vi "Collection.Dialog.vi"(8 "error in (no error)":errorcluster, 9 "ID":u16=1 min=1 format="%.0x", 10 "Existing PIDs":string[](array[string]), 11 "Name":string) -> (0 "error out":errorcluster, 1 "ID out":u16, 2 "Cancel PID?":bool, 3 "Name out":string)   [LabVIEW 2024, in "Diagnostics Addon System Explorer.lvlib"]
uses:
  Diagnostics Addon System Explorer.lvlib
  <vilib>/NI/AMC/Create Single Message.vi
  <vilib>/NI/AMC/Update Message Routing Info.vi
  <vilib>/NI/AMC/Read Termination Message.vi
  <vilib>/NI/AMC/Globals.vi
  <vilib>/NI/AMC/Send Message.vi
  <vilib>/NI/AMC/AMC.lvlib
panel:
  in  "Cancel PID":bool
  in  "Apply":bool
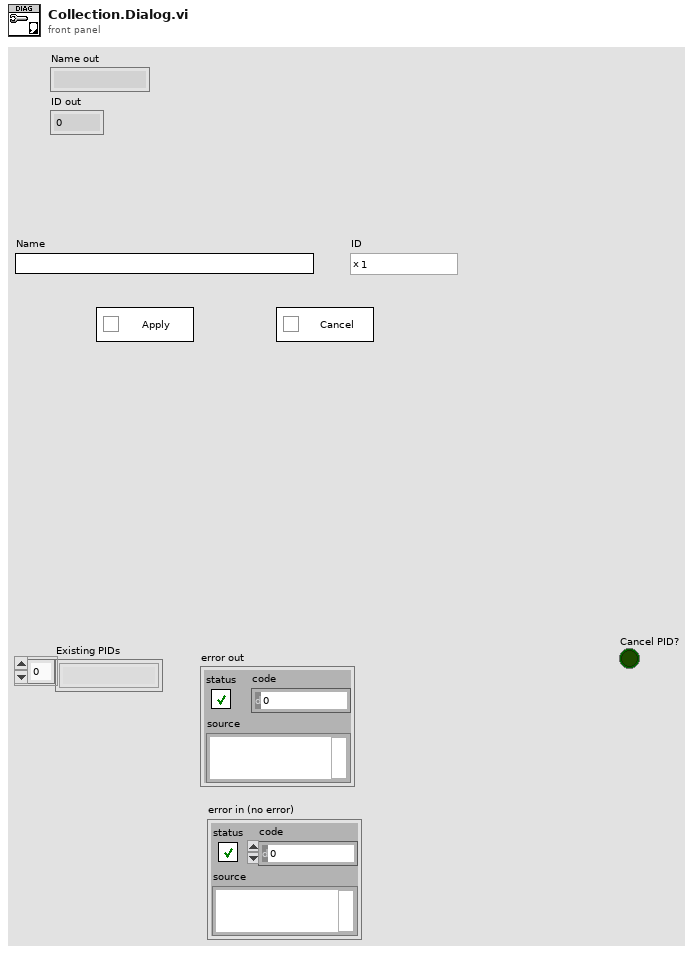
[diagram p1: front panel]
types:
  T1 = cluster{"Apply":refnum<vi>, "Cancel PID":refnum<vi>}
  T2 = typedef "AMC.lvlib/Message Queue.ctl" = refnum<queue>
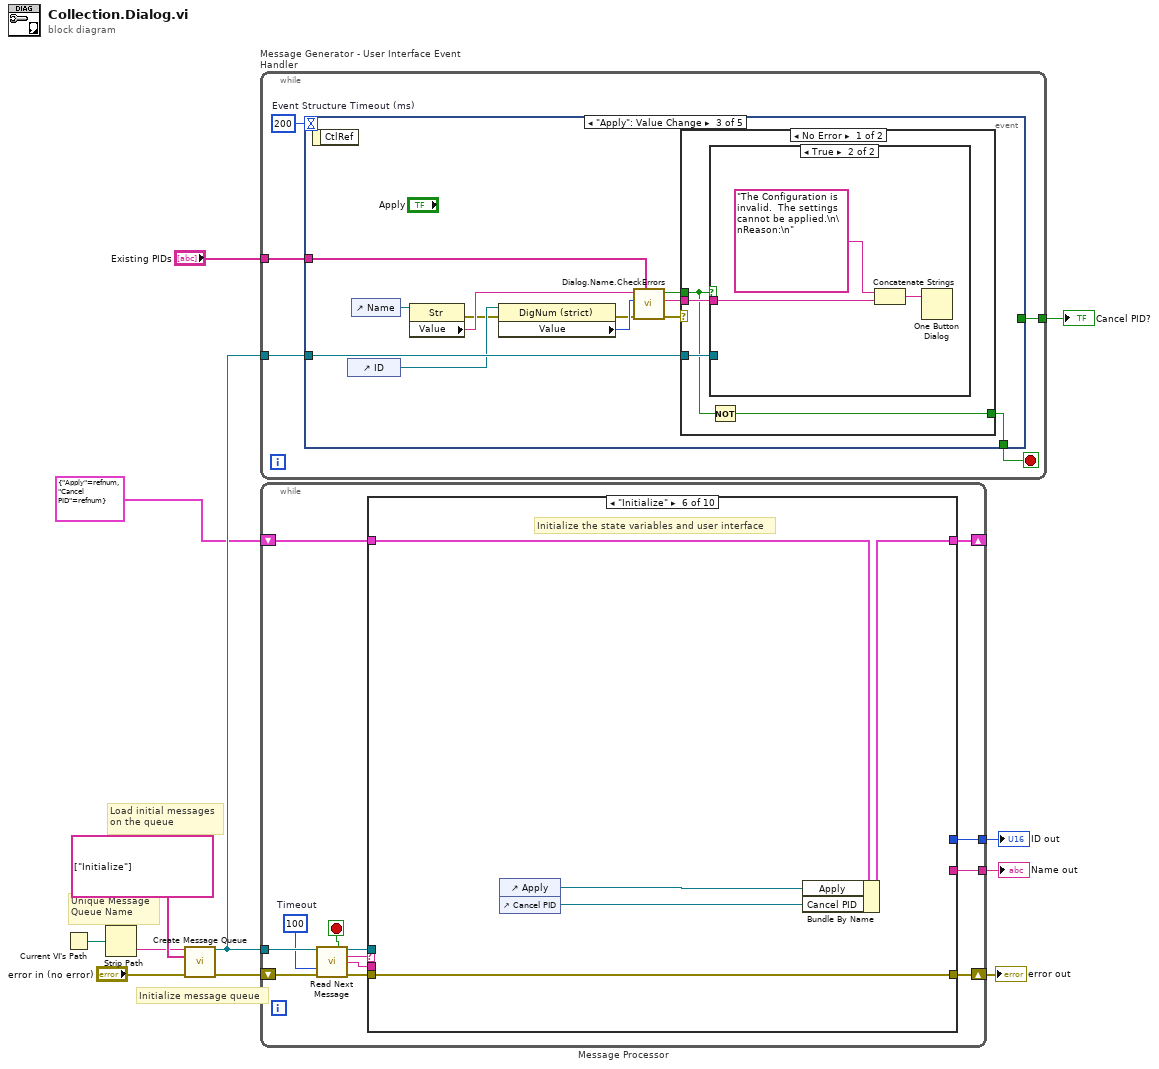
[diagram p0: block diagram]
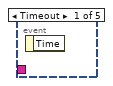
[diagram p2: hidden frame]
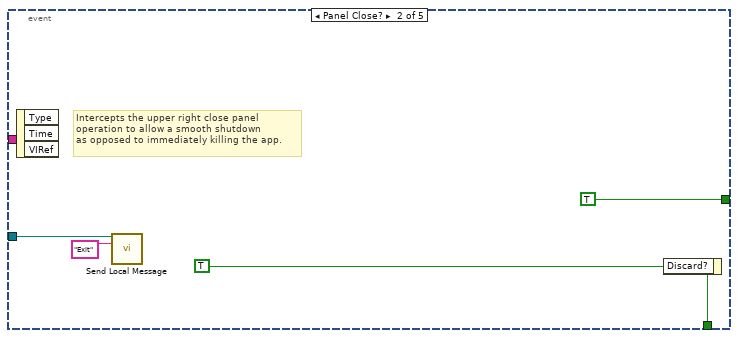
[diagram p3: hidden frame]
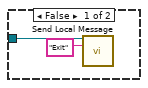
[diagram p4: hidden frame]
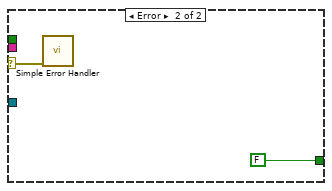
[diagram p5: hidden frame]
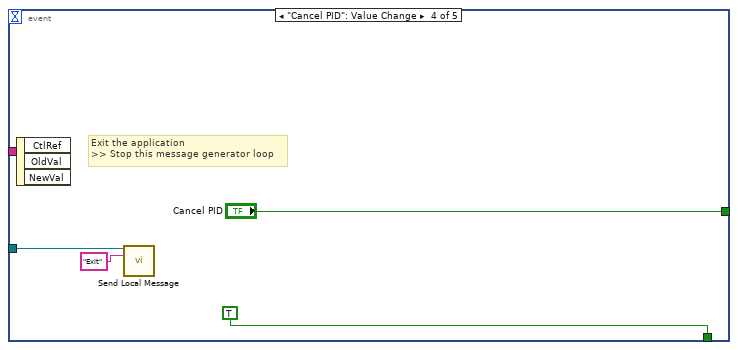
[diagram p6: hidden frame]
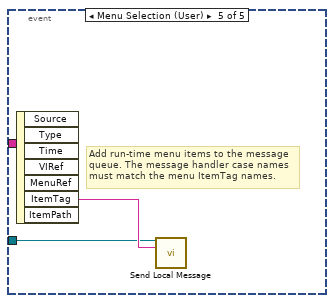
[diagram p7: hidden frame]
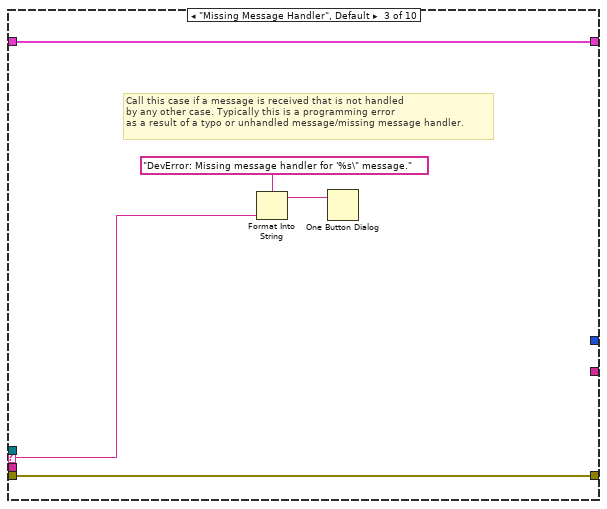
[diagram p10: hidden frame]
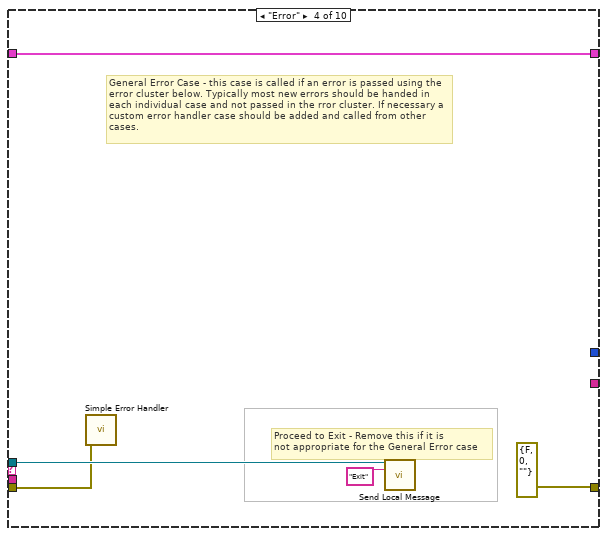
[diagram p11: hidden frame]
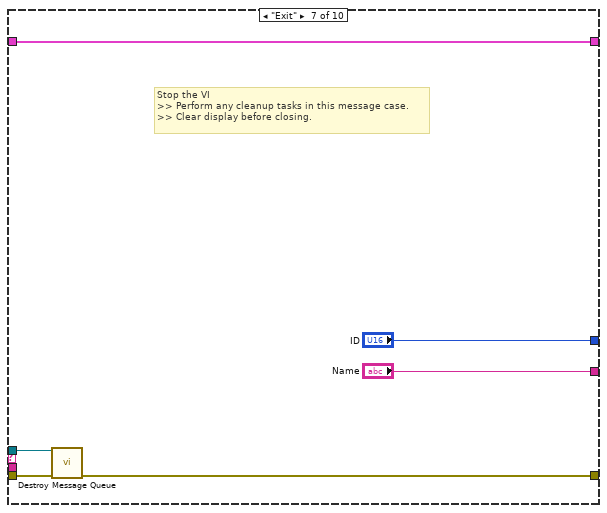
[diagram p13: hidden frame]
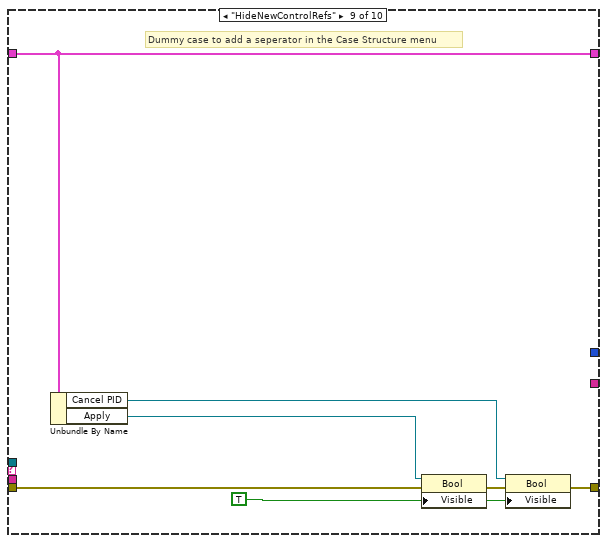
[diagram p15: hidden frame]
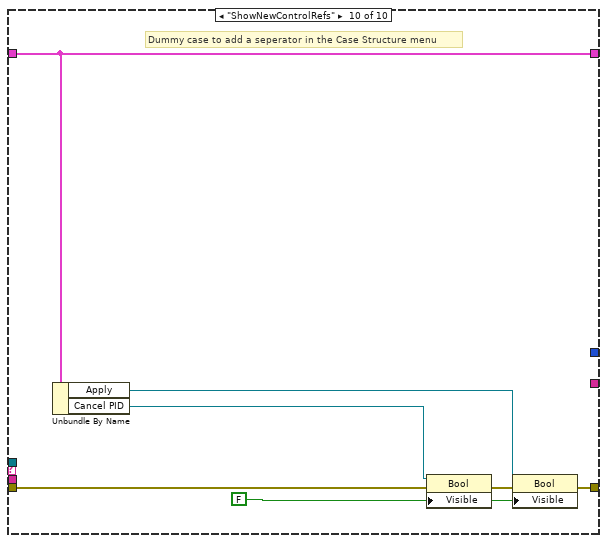
[diagram p16: hidden frame]
diagram:
  # "Initialize message queue"
  # "Unique Message\nQueue Name"
  # "Load initial messages\non the queue"
  n1 = Current VI's Path() -> (path=w8:path)
  n2 = Strip Path(path=w8) -> (name=w11:string)  [unwired: 1 out]
  n3 = call <vilib>:"Create Message Queue.vi"("message queue name"=w11, "initial message names"=string[] ["Initialize"], "error in"="error in (no error)") -> ("message queue out"=w10:T2, "error out"=w9:errorcluster)  [unwired: 11 in]
  n4 = while "Message Generator - User Interface Event Handler" {
    tunnel: w10 -> [w15]
    tunnel: [w14] -> w6
    tunnel: "Existing PIDs" -> [w13]
    stop <- w16 stop-if-true
    w17 = 200  # Event Structure Timeout (ms)
    n5 = event shown="[2] \"Apply\": Value Change" {
      selector: _ -> [_ _ _ _ _]
      dyn-events: _ -> [_ _ _ _ _]
      timeout: w17 -> [_ _ _ _ _]
      tunnel: [_ w21 w32 TRUE ("Discard?") _] -> w16
      tunnel: w15 -> [_ w19 w33 w46 w49]
      tunnel: [_ TRUE ("Cancel PID") _ "Cancel PID" _] -> w14
      tunnel: w13 -> [_ _ w28 _ _]
      event Timeout {
        n6 = event-data() -> ()  [unwired: 2 out]
      }
      event Panel Close? {
        w21 = TRUE ("Discard?")
        # "Intercepts the upper right close panel\noperation to allow a smooth shutdown\nas opposed to immediately killing the app."
        n7 = event-data() -> ()  [unwired: 4 out]
        n8 = call <vilib>:"Send Local Message.vi"("message queue in"=w19, "message name"="Exit") -> ()  [unwired: 11 in, 3 out]
        n9 = event-data("Discard?"=w21) -> ()  [unwired: 1 in, 1 out]
      }
      event "Apply": Value Change {
        n10 = event-data() -> ()  [unwired: 2 out]
        n11 = control-ref of="ID"() -> (w26:refnum<vi>)
        n12 = control-ref of="Name"() -> (w27:refnum<vi>)
        n13 = property class="Str"(reference=w27) -> (error out=w22:errorcluster, "Value"=w24:string)  [unwired: 1 in, 1 out]
        n14 = property class="DigNum (strict)"(reference=w26, error in=w22) -> (error out=w23:errorcluster, "Value"=w25:u16)  [unwired: 1 out]
        n15 = call "Dialog.Name.CheckErrors.vi"("Existing Frames"=w28, "error in (no error)"=w23, "ID"=w25, "Name"=w24) -> ("error out"=w31:errorcluster, "Error"=w29:string, "Error?"=w30:bool)  [unwired: 5 in]
        n16 = case shown="No Error" w31 {
          selector: w31 -> [_ w44]
          tunnel: w30 -> [w35 _]
          tunnel: w33 -> [w37 _]
          tunnel: w29 -> [w36 _]
          tunnel: [w34 FALSE] -> w32
          frame No Error {
            n17 = case shown="True" w35 {
              tunnel: w37 -> [w39 _]
              tunnel: w36 -> [_ w42]
              frame False {
                n18 = call <vilib>:"Send Local Message.vi"("message queue in"=w39, "message name"="Exit" ("Message Name")) -> ()  [unwired: 11 in, 3 out]
              }
              frame True {
                n19 = Concatenate Strings("The Configuration is invalid.  The settings cannot be applied.\n\nReason:\n" ("message"), w42) -> (w40:string)
                n20 = One Button Dialog(message=w40) -> ()  [unwired: 1 in, 1 out]
              }
            }
            n21 = Not(x=w35) -> (.not. x?=w34:bool)
          }
          frame Error {
            n22 = call <vilib>:"Simple Error Handler.vi"("error in (no error)"=w44) -> ()  [unwired: 4 in, 5 out]
          }
        }
      }
      event "Cancel PID": Value Change {
        # "Exit the application\n>> Stop this message generator loop"
        n23 = event-data() -> ()  [unwired: 4 out]
        n24 = call <vilib>:"Send Local Message.vi"("message queue in"=w46, "message name"="Exit") -> ()  [unwired: 11 in, 3 out]
      }
      event Menu Selection (User) {
        # "Add run-time menu items to the message\nqueue. The message handler case names must match the menu ItemTag names."
        n25 = event-data() -> ("ItemTag"=w50:string)  [unwired: 7 out]
        n26 = call <vilib>:"Send Local Message.vi"("message queue in"=w49, "message name"=w50) -> ()  [unwired: 11 in, 3 out]
      }
    }
  }
  "Cancel PID?" <- w6
  n27 = while "Message Processor" {
    shift-left: w9 -> [w57]
    shift-right: [w61] -> w4
    tunnel: w10 -> [w58]
    shift-left: T1 {"Apply"=refnum, "Cancel PID"=refnum} ("State Variables") -> [w63]
    shift-right: [w62] -> _
    tunnel: [w52] -> w2
    tunnel: [w51] -> w1
    stop <- w60 stop-if-true
    w55 = 100  # Timeout
    n28 = call <vilib>:"Read Next Message.vi"("message queue in"=w58, "timeout (1 ms)"=w55, "error in"=w57) -> ("exit process?"=w60:bool, "message queue out"=w59:T2, "message name"=w54:string, "message value"=w53:string, "error out"=w56:errorcluster)  [unwired: 5 in, 3 out]
    n29 = case shown="\"Initialize\"" w54 {
      selector: w54 -> [_ _ w70 _ _ _ _ _ _ _]
      tunnel: [w65 w67 w72 w77 w79 w83 w88 w92 w99 w106] -> w62
      tunnel: w63 -> [w65 w67 w72 w77 w79 w84 w88 w92 w99 w106]
      tunnel: w59 -> [_ _ _ w75 _ _ w89 _ _ _]
      tunnel: w56 -> [w64 w66 w71 w73 w78 w82 w90 w91 w93 w100]
      tunnel: [w64 w66 w71 errorcluster {"status"=FALSE, "code"=0, "source"=""} ("error out") w78 w82 w87 w91 w96 w104] -> w61
      tunnel: w53 -> [_ _ _ _ _ _ _ _ _ _]
      tunnel: [_ _ _ _ _ _ "Name" _ _ _] -> w52
      tunnel: [_ _ _ _ _ _ "ID" _ _ _] -> w51
      frame "---------- Framework Operations ----------" {
        # "Dummy case to add a seperator in the Case Structure menu"
      }
      frame "", "Idle" {
        # "Idle Case - this case is called after a Timeout on the Get Next Message from Queue VI, if no new messages are present on the queue. This case can be used for housekeeping tasks such as updating the UI."
      }
      frame "Missing Message Handler", Default {
        # "Call this case if a message is received that is not handled \nby any other case. Typically this is a programming error\nas a result of a typo or unhandled message/missing message handler."
        n30 = Format Into String(format string="DevError: Missing message handler for '%s\" message." ("message"), w70) -> (resulting string=w68:string)  [unwired: 2 in, 1 out]
        n31 = One Button Dialog(message=w68) -> ()  [unwired: 2 out]
      }
      frame "Error" {
        # "Proceed to Exit - Remove this if it is\nnot appropriate for the General Error case"
        # "General Error Case - this case is called if an error is passed using the error cluster below. Typically most new errors should be handed in each individual case and not passed in the rror cluster. If necessary a custom error handler case should be added and called from other cases."
        n32 = call <vilib>:"Simple Error Handler.vi"("error in (no error)"=w73) -> ()  [unwired: 1 in, 8 out]
        n33 = call <vilib>:"Send Local Message.vi"("message queue in"=w75, "message name"="Exit") -> ()  [unwired: 11 in, 3 out]
      }
      frame "---------- Generic Operations ----------" {
        # "Dummy case to add a seperator in the Case Structure menu"
      }
      frame "Initialize" {
        # "Initialize the state variables and user interface"
        n34 = control-ref of="Apply"() -> (w81:refnum<vi>)
        n35 = control-ref of="Cancel PID"() -> (w80:refnum<vi>)
        n36 = Bundle By Name(cluster=w84, "Apply"=w81, "Cancel PID"=w80) -> (w83:T1)
      }
      frame "Exit" {
        # "Stop the VI\n>> Perform any cleanup tasks in this message case.\n>> Clear display before closing."
        n37 = call <vilib>:"Destroy Message Queue.vi"("message queue in"=w89, "error in"=w90) -> ("error out"=w87:errorcluster)  [unwired: 11 in, 2 out]
      }
      frame "---------- Application Operations ----------" {
        # "Dummy case to add a seperator in the Case Structure menu"
      }
      frame "HideNewControlRefs" {
        w97 = TRUE ("Visible")
        # "Dummy case to add a seperator in the Case Structure menu"
        n38 = Unbundle By Name(w99) -> ("Cancel PID"=w94:refnum<vi>, "Apply"=w95:refnum<vi>)
        n39 = property class="Bool"(reference=w95, error in=w93, "Visible"=w97) -> (error out=w98:errorcluster)  [unwired: 1 out]
        n40 = property class="Bool"(reference=w94, error in=w98, "Visible"=w97) -> (error out=w96:errorcluster)  [unwired: 1 out]
      }
      frame "ShowNewControlRefs" {
        w103 = FALSE ("Visible")
        # "Dummy case to add a seperator in the Case Structure menu"
        n41 = Unbundle By Name(w106) -> ("Apply"=w102:refnum<vi>, "Cancel PID"=w101:refnum<vi>)
        n42 = property class="Bool"(reference=w101, error in=w100, "Visible"=w103) -> (error out=w105:errorcluster)  [unwired: 1 out]
        n43 = property class="Bool"(reference=w102, error in=w105, "Visible"=w103) -> (error out=w104:errorcluster)  [unwired: 1 out]
      }
    }
  }
  "error out" <- w4
  "Name out" <- w2
  "ID out" <- w1
